vi "Utilities.Buffer.Double.vi"(8 "error in (no error)":errorcluster, 10 "buffer in":dbl[](array[numeric]), 11 "minimum size":i64) -> (0 "error out":errorcluster, 2 "buffer out":dbl[](array[numeric]))   [LabVIEW 2016, in "VeriStand Data.lvlib"]
uses:
  VeriStand Data.lvlib
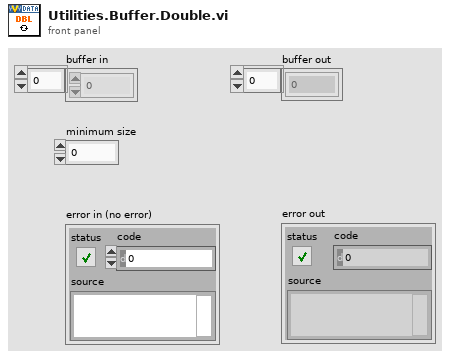
[diagram p1: front panel]
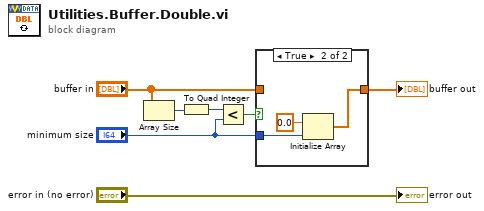
[diagram p0: block diagram]
diagram:
  n1 = Array Size(array="buffer in") -> (size(s)=w6:i32)
  n2 = To Quad Integer(1:w6) -> (0:w1:i64)
  n3 = Less?(x=w1, y="minimum size") -> (x < y?=w4:bool)
  n4 = case shown="True" w4 {
    tunnel: "buffer in" -> [w8 _]
    tunnel: "minimum size" -> [_ w10]
    tunnel: [w8 w9] -> w3
    frame False {
    }
    frame True {
      n5 = Initialize Array(0.0 ("element"), w10) -> (w9:dbl[])
    }
  }
  "buffer out" <- w3
  "error out" <- "error in (no error)"
